vi "CAN Initialize FD.vi"(8 "error in (no error)":errorcluster, 10 "BitrateFD":string, 11 "Channel":u16) -> (0 "error out":errorcluster, 2 "BitrateFD out":string, 3 "function return":u32)   [LabVIEW 2017, in "PCANBasic_eX.lvlib"]
doc: "TPCANStatus __stdcall CAN_InitializeFD(\n TPCANHandle Channel,\n TPCANBitrateFD BitrateFD);"
uses:
  PCANBasic_eX.lvlib
  PCANBasic.dll
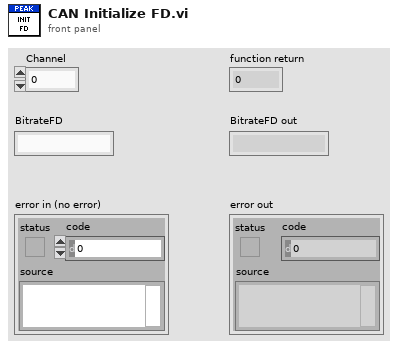
[diagram p1: front panel]
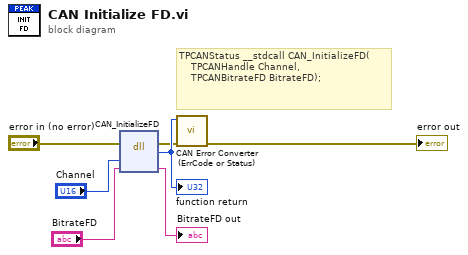
[diagram p0: block diagram]
diagram:
  # "TPCANStatus __stdcall CAN_InitializeFD(\n    TPCANHandle Channel,\n\t   TPCANBitrateFD BitrateFD);"
  n1 = dll-call lib="PCANBasic.*" fn="CAN_InitializeFD"(error in="error in (no error)", "Channel"="Channel", "BitrateFD"="BitrateFD") -> (error out=w2:errorcluster, w7:u32, "BitrateFD"=→"BitrateFD out":string)  [unwired: 3 in, 1 out]
  "function return" <- w7
  n2 = call "CAN Error Converter (ErrCode or Status).vi"("error in (no error)"=w2, "error code"=w7) -> ("error out"=→"error out":errorcluster)  [unwired: 9 in]
